vi "GetDefaultParams.vi"(8 "error in (no error)":errorcluster, 10 "Path":path, 11 "ArbitraryFunction.lvclass":refnum<class "ArbitraryFunction.lvclass">) -> (0 "error out":errorcluster, 3 "ArbitraryFunction.lvclass":refnum<class "ArbitraryFunction.lvclass">)   [LabVIEW 2014, in "Functions.lvlib" / "ArbitraryFunction.lvclass"]
uses:
  ArbitraryFunction.lvclass
  FunctionBaseClass/FunctionBase.lvclass/FunctionBase.ctl
  TypeDefs/Arbitrary.ctl
  ArbitraryFunction.lvclass/ArbitraryFunction.ctl
  FunctionBaseClass/Accessors/Read FunctionIniFilePath.vi
  Accessors/Write SampleRate.vi
  Accessors/Write Arbs.vi
  Accessors/Write Count.vi
  FunctionBaseClass/FunctionBase.lvclass
  <vilib>/Utility/config.llb/NI_LVConfig.lvlib
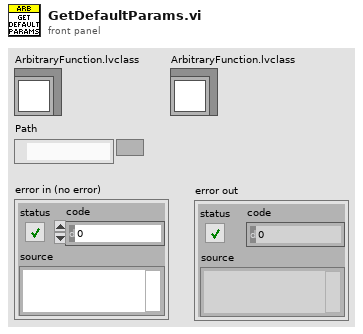
[diagram p1: front panel]
types:
  T1 = cluster{"Handle":string, "Size":i32, "Gain":dbl, "Offset":dbl}[]
  T2 = typedef "NI_LVConfig.lvlib/Config Data RefNum.ctl" = refnum<k1>
  T3 = typedef "Functions.lvlib/ArbitraryFunction.lvclass/Arbitrary.ctl" = cluster{"Handle":string, "Size":i32, "Gain":dbl, "Offset":dbl, "Waveform":waveform(dbl)}
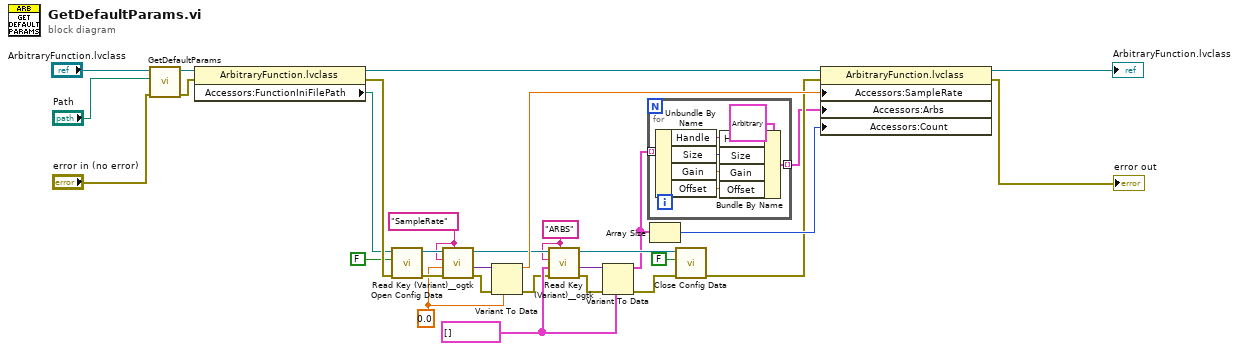
[diagram p0: block diagram]
diagram:
  w13 = T1 [] ("Arbs")
  w3 = "ARBS" ("section")
  w16 = 0.0 ("SampleRate")
  w19 = "SampleRate" ("section")
  n1 = call-parent "GetDefaultParams.vi"("error in (no error)"="error in (no error)", "Path"="Path", "FunctionBase in"="ArbitraryFunction.lvclass") -> ("error out"=w26:errorcluster, "FunctionBase out"=w30:refnum<class "ArbitraryFunction.lvclass">)  [unwired: 7 in]
  n2 = property class="ArbitraryFunction.lvclass"(reference=w30, error in=w26) -> (reference out=w27:refnum<class "ArbitraryFunction.lvclass">, error out=w24:errorcluster, "Accessors:FunctionIniFilePath"=w23:path)
  n3 = call <vilib>:"Open Config Data.vi"("error in (no error)"=w24, "create file if necessary (T)"=FALSE, "configuration file path"=w23) -> ("error out"=w21:errorcluster, "refnum"=w20:T2)  [unwired: 6 in, 1 out]
  n4 = call <userlib>:"Read Key (Variant)__ogtk.vi"("section"=w19, "error in (no error)"=w21, "type"=w16, "key (optional)"=w19, "refnum"=w20) -> ("error out"=w17:errorcluster, "key-value"=w18:variant, "refnum out"=w14:T2)  [unwired: 3 in, 1 out]
  n5 = Variant To Data(error in=w17, type=w16, Variant=w18) -> (data=w15:dbl, error out=w11:errorcluster)
  n6 = call <userlib>:"Read Key (Variant)__ogtk.vi"("section"=w3, "error in (no error)"=w11, "type"=w13, "key (optional)"=w3, "refnum"=w14) -> ("error out"=w10:errorcluster, "key-value"=w12:variant, "refnum out"=w7:T2)  [unwired: 3 in, 1 out]
  n7 = Variant To Data(error in=w10, type=w13, Variant=w12) -> (data=w2:T1, error out=w6:errorcluster)
  n8 = for {
    tunnel: w2 -> [w37] mode=indexing
    tunnel: [w32] -> w1 mode=indexing
    n9 = Unbundle By Name(w37) -> ("Handle"=w33:string, "Size"=w34:i32, "Gain"=w35:dbl, "Offset"=w36:dbl)
    n10 = Bundle By Name(cluster=T3 {"Handle"="", "Size"=0, "Gain"=0.0, "Offset"=0.0, "Waveform"={"t0"=timestamp(0 s since 1904-01-01), "dt"=1.0, "Y"=[]}} ("Arbitrary"), "Handle"=w33, "Size"=w34, "Gain"=w35, "Offset"=w36) -> (w32:T3)
  }
  n11 = Array Size(array=w2) -> (size(s)=w9:i32)
  n12 = call <vilib>:"Close Config Data.vi"("error in (no error)"=w6, "write file if changed (T)"=FALSE, "refnum"=w7) -> ("error out"=w4:errorcluster)  [unwired: 7 in, 1 out]
  n13 = property class="ArbitraryFunction.lvclass"(reference=w27, error in=w4, "Accessors:SampleRate"=w15, "Accessors:Arbs"=w1, "Accessors:Count"=w9) -> (reference out=→"ArbitraryFunction.lvclass":refnum<class "ArbitraryFunction.lvclass">, error out=→"error out":errorcluster)
